vi "DB-Schema.vi"() -> (0 "DB Schema (public.)":string)   [LabVIEW 2016, in "DB-Configuration.lvlib"]
doc: "Name of database schema, e.g. \"public.\"\n\nEdit the schema constant to your needs."
uses:
  DB-Configuration.lvlib
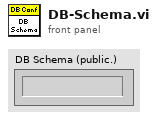
[diagram p1: front panel]
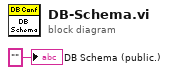
[diagram p0: block diagram]
diagram:
  "DB Schema (public.)" <- "" ("DB Table Prefix")
